vi "Spinner.vi"(5 "Enum":enum16{"Spinner 1", "Spinner 2", "Spinner 3"}(ring)) -> (2 "Spinner Out":string="(-*--------)")   [LabVIEW 2019, in "Instrument UI.Lockin.lvclass"]
uses:
  Instrument UI.Lockin.lvclass
panel:
  in  "Spinner 2":string="    \n.   \n..  \n... \n....\n... \n..  \n.   "
  in  "Spinner 1":string="(*---------)\n(-*--------)\n(--*-------)\n(---*------)\n(----*-----)\n(-----*----)\n(------*---)\n(-------*--)\n(--------*-)\n(---------*)\n(--------*-)\n(-------*--)\n(------*---)\n(-----*----)\n(----*-----)\n(---*------)\n(--*-------)\n(-*--------)"
  in  "spinner 3":string=" /\n--\n \\\n |\n /\n--\n \\\n |"
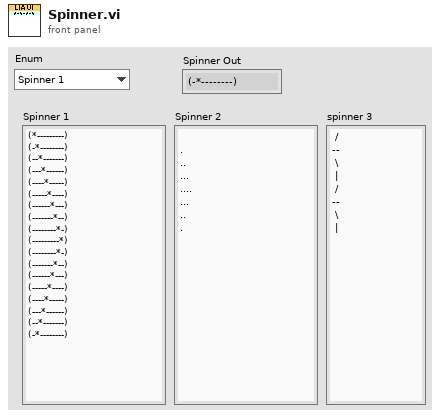
[diagram p1: front panel]
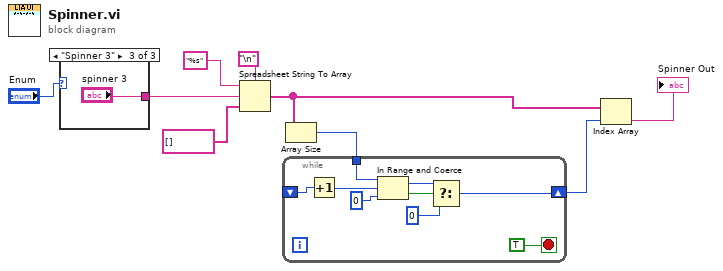
[diagram p0: block diagram]
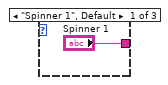
[diagram p2: hidden frame]
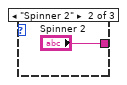
[diagram p3: hidden frame]
diagram:
  n1 = case shown="\"Spinner 3\"" "Enum" {
    tunnel: ["Spinner 1" "Spinner 2" "spinner 3"] -> w1
    frame "Spinner 1", Default {
    }
    frame "Spinner 2" {
    }
    frame "Spinner 3" {
    }
  }
  n2 = Spreadsheet String To Array(delimiter (Tab)="\n", format string="%s", spreadsheet string=w1, array type (2D Dbl)=string[] []) -> (array=w6:string[])
  n3 = Array Size(array=w6) -> (size(s)=w5:i32)
  n4 = while {
    shift-right: [w15] -> w7
    shift-left: _ -> [w21]
    tunnel: w5 -> [w13]
    stop <- TRUE stop-if-true
    n5 = Increment(x=w21) -> (x+1=w17:u32)
    n6 = In Range and Coerce(upper limit=w13, x=w17, lower limit=u32 0) -> (coerced(x)=w18:u32, In Range?=w19:bool)
    n7 = Select(t=w18, s=w19, f=u32 0) -> (s? t:f=w15:u32)
  }
  n8 = Index Array(array=w6, index=w7) -> (element=→"Spinner Out":string)
